vi "E710_Sample_Application_1.vi"() -> ()   [LabVIEW 2011]
doc: "This VI demonstrates how to statically define an E-710 configuration with one connected axis. In this example the E-710 is connected through COM port 1 with baudrate 57600. The VI runs E710_Configuration_Setup.vi with these specified settings, performs an automated zero-point calibration of the connected axis and reads the position of the axis. The diagram shows how to combine the driver VIs for these tasks. \n\nWarning: Before running this VI, modify the \"Interface\" and \"RS232 settings\" to reflect your configuration. The predefined settings provided with the VI probably do not match your system."
panel:
  in  "stop":bool
  out "ATZ successful?":bool[](array[boolean])
  in  "error in":errorcluster
  out "Running":bool caption="Axis is referencing"
  out "error out":errorcluster
  out "Position":dbl[](array[numeric]) format="%.6f"
  out "Conn. Axis":string[](array[string])
  out "Identification":string
  # "Simple E-710 sample program"
  # "This VI demonstrates how to statically define an E-710 configuration with one connected axis. In this example the E-710 is connected through COM port \n1 with baudrate 57600. The VI runs E710_Configuration_Setup.vi with these specified settings, performs an automated zero-point calibration of the \nconnected axis  and reads the position of the axis. The diagram shows how to combine the driver VIs for these tasks. \n\nWarning: Before running this VI, modify the \"Interface\" and \"RS232 settings\" to reflect your configuration. The predefined \n                 settings provided with the VI probably do not match your system."
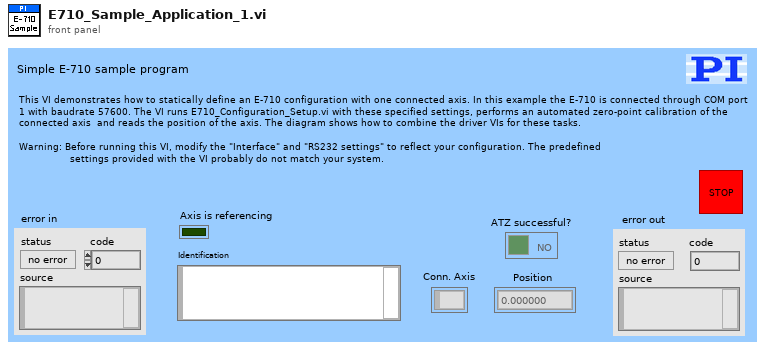
[diagram p1: front panel]
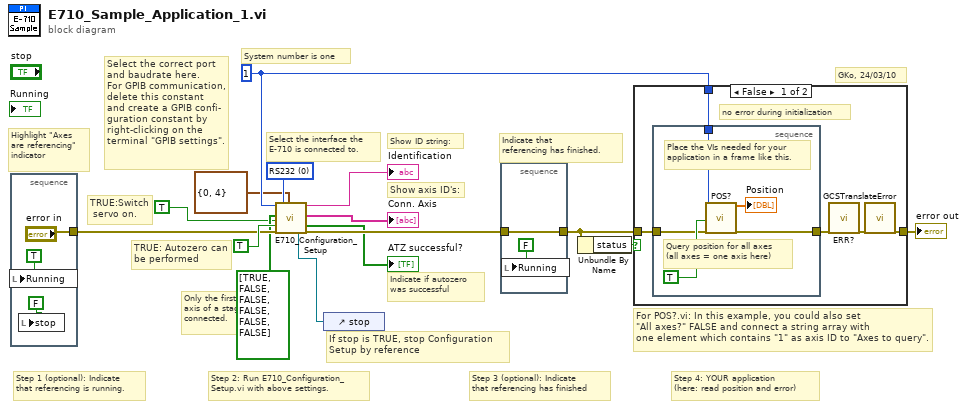
[diagram p0: block diagram]
diagram:
  w8 = u16 0 items=["RS232", "GPIB"] ("Interface")
  w13 = 1 ("System no.")
  # "TRUE:Switch\n servo on."
  # "If stop is TRUE, stop Configuration\nSetup by reference"
  # "Indicate if autozero \nwas successful"
  # "Only the first\naxis of a stage is\nconnected."
  # "Select the interface the\nE-710 is connected to."
  # "Select the correct port \nand baudrate here.\nFor GPIB communication, \ndelete this constant\nand create a GPIB confi-\nguration constant by\nright-clicking on the \nterminal \"GPIB settings\"."
  # "GKo, 24/03/10"
  # "Step 4: YOUR application\n(here: read position and error)"
  # "Step 3 (optional): Indicate\nthat referencing has finished"
  # "Step 2: Run E710_Configuration_\nSetup.vi with above settings."
  # "Step 1 (optional): Indicate\nthat referencing is running."
  # "Indicate that\nreferencing has finished."
  # "Highlight \"Axes\nare referencing\"\nindicator"
  # "For POS?.vi: In this example, you could also set\n\"All axes?\" FALSE and connect a string array with \none element which contains \"1\" as axis ID to \"Axes to query\"."
  # "Show axis ID's:"
  # "Show ID string:"
  # "TRUE: Autozero can\nbe performed"
  # "System number is one"
  n1 = stacked-sequence {
    tunnel: ["error in"] -> w10
    frame #0 {
      n2 = local write "Running"(TRUE ("Running")) -> ()
      n3 = local write "stop"(FALSE ("stop")) -> ()
    }
  }
  n4 = control-ref of="stop"() -> (w3:refnum<vi>)
  n5 = call "E710_Configuration_Setup.vi"("System no."=w13, "Are stages connected?"=bool[] [TRUE, FALSE, FALSE, FALSE, FALSE, FALSE], "Change servo \nstatus to ON?"=TRUE ("Change servo \nstatus to ON?"), "Perform autozero?"=TRUE ("All axes?"), "error in"=w10, "Interface"=w8, "RS232 settings"=cluster{"Portnumber":i32, "Baudrate":u16} {"Portnumber"=0, "Baudrate"=4}, "Stop refnum"=w3) -> ("Identification"=→"Identification":string, "Conn. Axes"=→"Conn. Axis":string[], "ATZ successful?"=→"ATZ successful?":bool[], "error out"=w11:errorcluster)  [unwired: 4 in, 4 out]
  n6 = stacked-sequence {
    tunnel: w11 -> [w20]
    tunnel: [w20] -> w5
    frame #0 {
      n7 = local write "Running"(FALSE ("Running")) -> ()
    }
  }
  n8 = Unbundle By Name(w5) -> ("status"=w4:bool)
  n9 = case shown="False" w4 {
    tunnel: w13 -> [w25 _]
    tunnel: [w21 w31] -> w12
    tunnel: w5 -> [w24 w31]
    frame False {
      # "no error during initialization"
      n10 = stacked-sequence {
        tunnel: w25 -> [w30]
        tunnel: w24 -> [w27]
        tunnel: [w26] -> w23
        frame #0 {
          # "Place the VIs needed for your\napplication in a frame like this."
          # "Query position for all axes\n(all axes = one axis here)"
          n11 = call "POS?.vi"("System no."=w30, "All axes?"=TRUE, "error in"=w27) -> ("Position"=→"Position":dbl[], "error out"=w26:errorcluster)  [unwired: 2 in, 13 out]
        }
      }
      n12 = call "ERR?.vi"("error in"=w23) -> ("error out"=w22:errorcluster)  [unwired: 1 in, 17 out]
      n13 = call "GCSTranslateError.vi"("error in"=w22) -> ("error out"=w21:errorcluster)  [unwired: 18 out]
    }
    frame True {
      # "Error during initialization,\nstop execution here."
    }
  }
  "error out" <- w12
